vi "Acquire.vi"(8 "error in (no error)":errorcluster, 10 "Message Queues":T1, 11 "Hardware Resources in":T4 {"Reference Distance" format="%.3g"}) -> (0 "error out":errorcluster, 2 "Message Queues out":T1, 3 "Hardware Resources out":T4 {"Reference Distance" format="%.3g"})   [LabVIEW 2018, in "Acquisition.lvlib"]
doc: "Perform the acquisition. Replace the contents of this diagram with calls to acquisition hardware."
uses:
  Acquisition.lvlib
  Hardware Configuration.ctl
  Support/Message Queue/All Message Queues.ctl
  Support/Message Queue/Message Cluster.ctl
  Controls/Data Queue.ctl
  Controls/Acquired Data.ctl
  Controls/Data Notifier.ctl
  support/Message Queue/Message Queue.lvlib
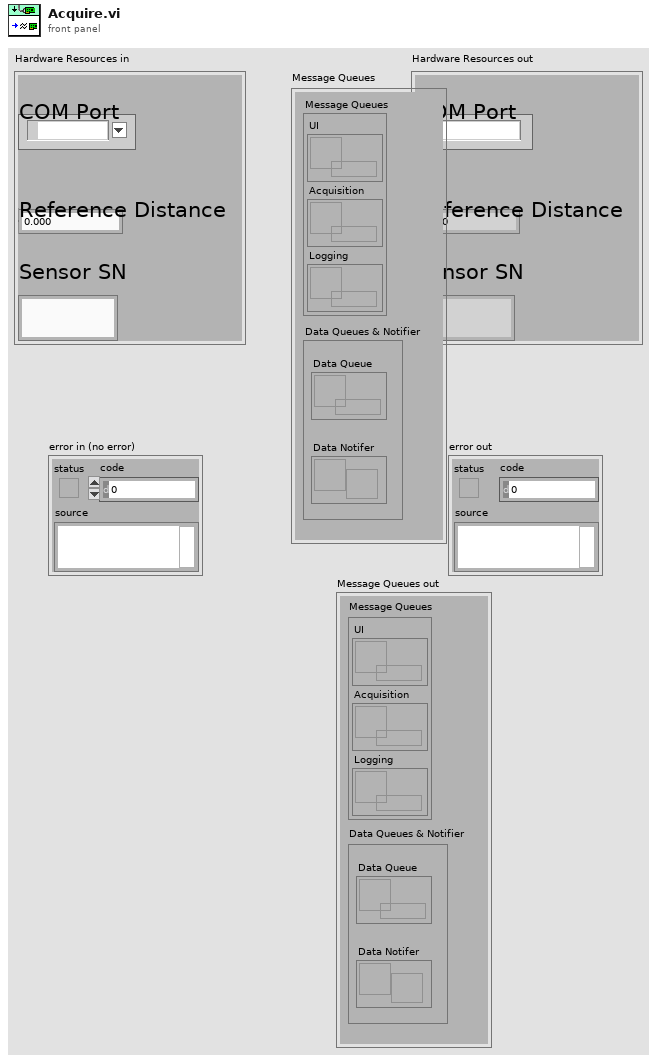
[diagram p1: front panel]
types:
  T1 = typedef "Message Queue.lvlib/All Message Queues.ctl" = cluster{"Message Queues":cluster{"UI":refnum<queue>, "Acquisition":refnum<queue>, "Logging":refnum<queue>}, "Data Queues & Notifier":cluster{"Data Queue":T2, "Data Notifer":T3}}
  T2 = typedef "Data Queue.ctl" = refnum<queue>
  T3 = typedef "Data Notifier.ctl" = refnum<notifier>
  T4 = typedef "Acquisition.lvlib/Hardware Configuration.ctl" = cluster{"COM Port":refnum<visa-resource-name>, "Reference Distance":dbl, "Sensor SN":string}
  T5 = typedef "Acquired Data.ctl" = cluster{"offset":dbl, "time":string}
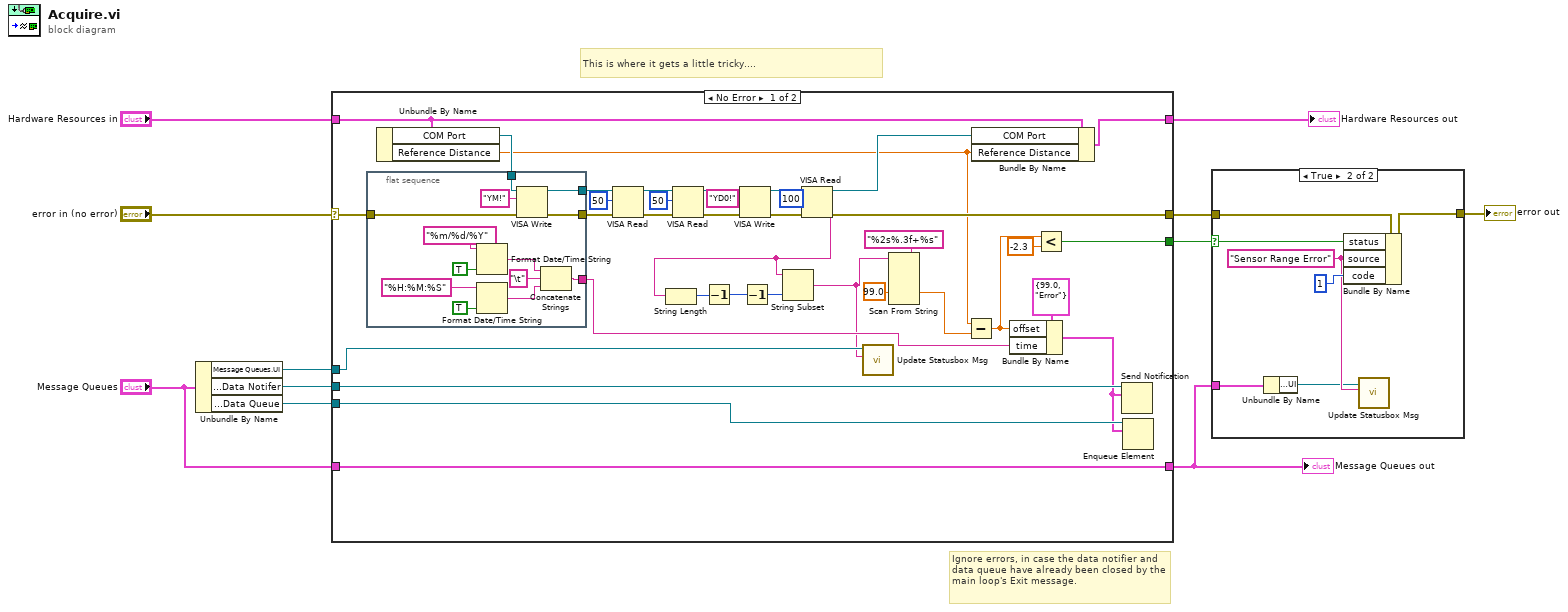
[diagram p0: block diagram]
diagram:
  # "Ignore errors, in case the data notifier and data queue have already been closed by the main loop's Exit message."
  # "This is where it gets a little tricky...."
  n1 = Unbundle By Name("Message Queues") -> ("Message Queues.UI"=w2:refnum<queue>, "Data Queues & Notifier.Data Notifer"=w8:T3, "Data Queues & Notifier.Data Queue"=w7:T2)
  n2 = case shown="No Error" "error in (no error)" {
    selector: "error in (no error)" -> [w28 w63]
    tunnel: [w27 w63] -> w4
    tunnel: "Hardware Resources in" -> [w47 w64]
    tunnel: [w48 w64] -> w9
    tunnel: w8 -> [w46 _]
    tunnel: w7 -> [w45 _]
    tunnel: "Message Queues" -> [w44 w62]
    tunnel: [w44 w62] -> w1
    tunnel: [w18 _] -> w5
    tunnel: w2 -> [w17 _]
    frame No Error {
      n3 = flat-sequence {
        tunnel: [w58] -> w36
        tunnel: [w57] -> w35
        tunnel: w29 -> [w56]
        tunnel: w28 -> [w55]
        tunnel: [w49] -> w21
        frame #0 {
          n4 = Format Date/Time String(time format string (%c)="%m/%d/%Y", UTC format=TRUE) -> (date/time string=w51:string)  [unwired: 1 in]
          n5 = Format Date/Time String(time format string (%c)="%H:%M:%S", UTC format=TRUE) -> (date/time string=w50:string)  [unwired: 1 in]
          n6 = VISA Write(VISA resource name=w56, write buffer="YM!", error in (no error)=w55) -> (VISA resource name out=w57:refnum<visa-resource-name>, error out=w58:errorcluster)  [unwired: 1 out]
          n7 = Concatenate Strings(w51, "\t", w50) -> (w49:string)
        }
      }
      n8 = Unbundle By Name(w47) -> ("COM Port"=w29:refnum<visa-resource-name>, "Reference Distance"=w24:dbl)
      n9 = VISA Read(VISA resource name=w35, byte count=u32 50, error in (no error)=w36) -> (VISA resource name out=w30:refnum<visa-resource-name>, error out=w33:errorcluster)  [unwired: 2 out]
      n10 = VISA Read(VISA resource name=w30, byte count=u32 50, error in (no error)=w33) -> (VISA resource name out=w31:refnum<visa-resource-name>, error out=w32:errorcluster)  [unwired: 2 out]
      n11 = VISA Write(VISA resource name=w31, write buffer="YD0!", error in (no error)=w32) -> (VISA resource name out=w43:refnum<visa-resource-name>, error out=w42:errorcluster)  [unwired: 1 out]
      n12 = VISA Read(VISA resource name=w43, byte count=u32 100, error in (no error)=w42) -> (VISA resource name out=w26:refnum<visa-resource-name>, read buffer=w15:string, error out=w27:errorcluster)  [unwired: 1 out]
      n13 = String Length(string=w15) -> (length=w16:i32)
      n14 = Decrement(x=w16) -> (x-1=w14:i32)
      n15 = Decrement(x=w14) -> (x-1=w13:i32)
      n16 = String Subset(string=w15, length (rest)=w13) -> (substring=w12:string)  [unwired: 1 in]
      n17 = call "Update Statusbox Msg.vi"("Message"=w12, "Queue in"=w17) -> ()  [unwired: 8 in, 2 out]
      n18 = Scan From String(format string="%2s%.3f+%s", input string=w12, default 2=99.0 ("default value 2")) -> (output 2=w25:dbl)  [unwired: 6 in, 3 out]
      n19 = Subtract(x=w24, y=w25) -> (x-y=w20:dbl)
      n20 = Bundle By Name(cluster=w47, "COM Port"=w26, "Reference Distance"=w24) -> (w48:T4)
      n21 = Bundle By Name(cluster=T5 {"offset"=99.0, "time"="Error"} ("notification"), "offset"=w20, "time"=w21) -> (w22:T5)
      n22 = Less?(x=w20, y=-2.3) -> (x < y?=w18:bool)
      n23 = Send Notification(notification=w22, notifier=w46) -> ()  [unwired: 1 in, 2 out]
      n24 = Enqueue Element(queue=w45, element=w22) -> ()  [unwired: 2 in, 3 out]
    }
    frame Error {
    }
  }
  "Hardware Resources out" <- w9
  "Message Queues out" <- w1
  n25 = case shown="True" w5 {
    selector: w5 -> [_ w70]
    tunnel: w4 -> [w65 w72]
    tunnel: [w65 w71] -> w3
    tunnel: w1 -> [_ w67]
    frame False {
    }
    frame True {
      w68 = "Sensor Range Error" ("source")
      n26 = Unbundle By Name(w67) -> ("Message Queues.UI"=w66:refnum<queue>)
      n27 = Bundle By Name(cluster=w72, "status"=w70, "source"=w68, "code"=1) -> (w71:errorcluster)
      n28 = call "Update Statusbox Msg.vi"("Message"=w68, "Queue in"=w66) -> ()  [unwired: 8 in, 2 out]
    }
  }
  "error out" <- w3
